vi "bias.vi"(10 "Cluster":T3={"Numero di punti"=11, "fattore-measdelay"=65, "Periodo"=0.01, "source autorange gate"=FALSE, "Tensione gate"=1.0, "llimit-gate"=1.0, "Source Function Gate"=1, "Range Mode Gate"=0, "Autozero Mode Gate"=1, "tensione drain"=1.0, "limit-drain"=1.0, "Autozero Mode Drain"=1, "Source Function Drain"=1, "Range Mode Drain"=0, "source autorange drain"=FALSE, "range-gate"=0.01, "source_range_gate"=2.0, "range-drain"=0.01, "source_range_drain"=2.0} {"source_range_drain" items=["200 mV"=0.2, "2 V"=2.0, "20 V"=20.0, "200 V"=200.0]; "range-drain" items=["100 nA"=1e-07, "1 uA"=1e-06, "10 uA"=1e-05, "100 uA"=0.0001, "1 mA"=0.001, "10 mA"=0.01, "100 mA"=0.1, "1 A"=1.0]; "source_range_gate" items=["200 mV"=0.2, "2 V"=2.0, "20 V"=20.0, "200 V"=200.0]; "range-gate" items=["100 nA"=1e-07, "1 uA"=1e-06, "10 uA"=1e-05, "100 uA"=0.0001, "1 mA"=0.001, "10 mA"=0.01, "100 mA"=0.1, "1 A"=1.0]; "Range Mode Drain" items=["Auto Range Off", "Auto Range On", "Auto Range Follow Limit"]; "Source Function Drain" items=["Current", "Voltage"]; "Autozero Mode Drain" items=["Autozero Off", "Autozero Once", "Autozero Auto"]; "limit-drain" format="%#_13g"; "Autozero Mode Gate" items=["Autozero Off", "Autozero Once", "Autozero Auto"]; "Range Mode Gate" items=["Auto Range Off", "Auto Range On", "Auto Range Follow Limit"]; "Source Function Gate" items=["Current", "Voltage"]; "llimit-gate" format="%#_13g"; "Periodo" items=["500 uS", "1 mS", "2 mS", "5 mS", "10 mS", "20 mS", "50 mS", "100 mS", "200 mS", "500 mS", "1 S", "2 S", "5 S", "10 S", ""]}, 11 "Cluster 3":T2={"VISA resource name out"="USB0::0x05E6::0x2612::4671051::INSTR", "error out"={"status"=FALSE, "code"=0, "source"=""}}) -> (2 "Cluster 2":T1, 3 "output cluster":T2)   [LabVIEW 2025]
uses:
  <instrlib>/Keithley 2600 Series/Keithley 2600 Series.lvlib
panel:
  out "range misurato gate":string
  out "range misurato drain":string
  out "finestra di misura":dbl
  out "measdelay":dbl
  out "Frequenza di rete (Hz)":dbl
  # "Impostazioni connessione"
  # "SMUA"
  # "SMUB"
  # "tabella valori"
  # "Impostazioni funzione source"
  # "Impostazioni comuni"
  # "GATE"
  # "DRAIN"
  # "Impostazioni funzione misura"
  # "GATE"
  # "DRAIN"
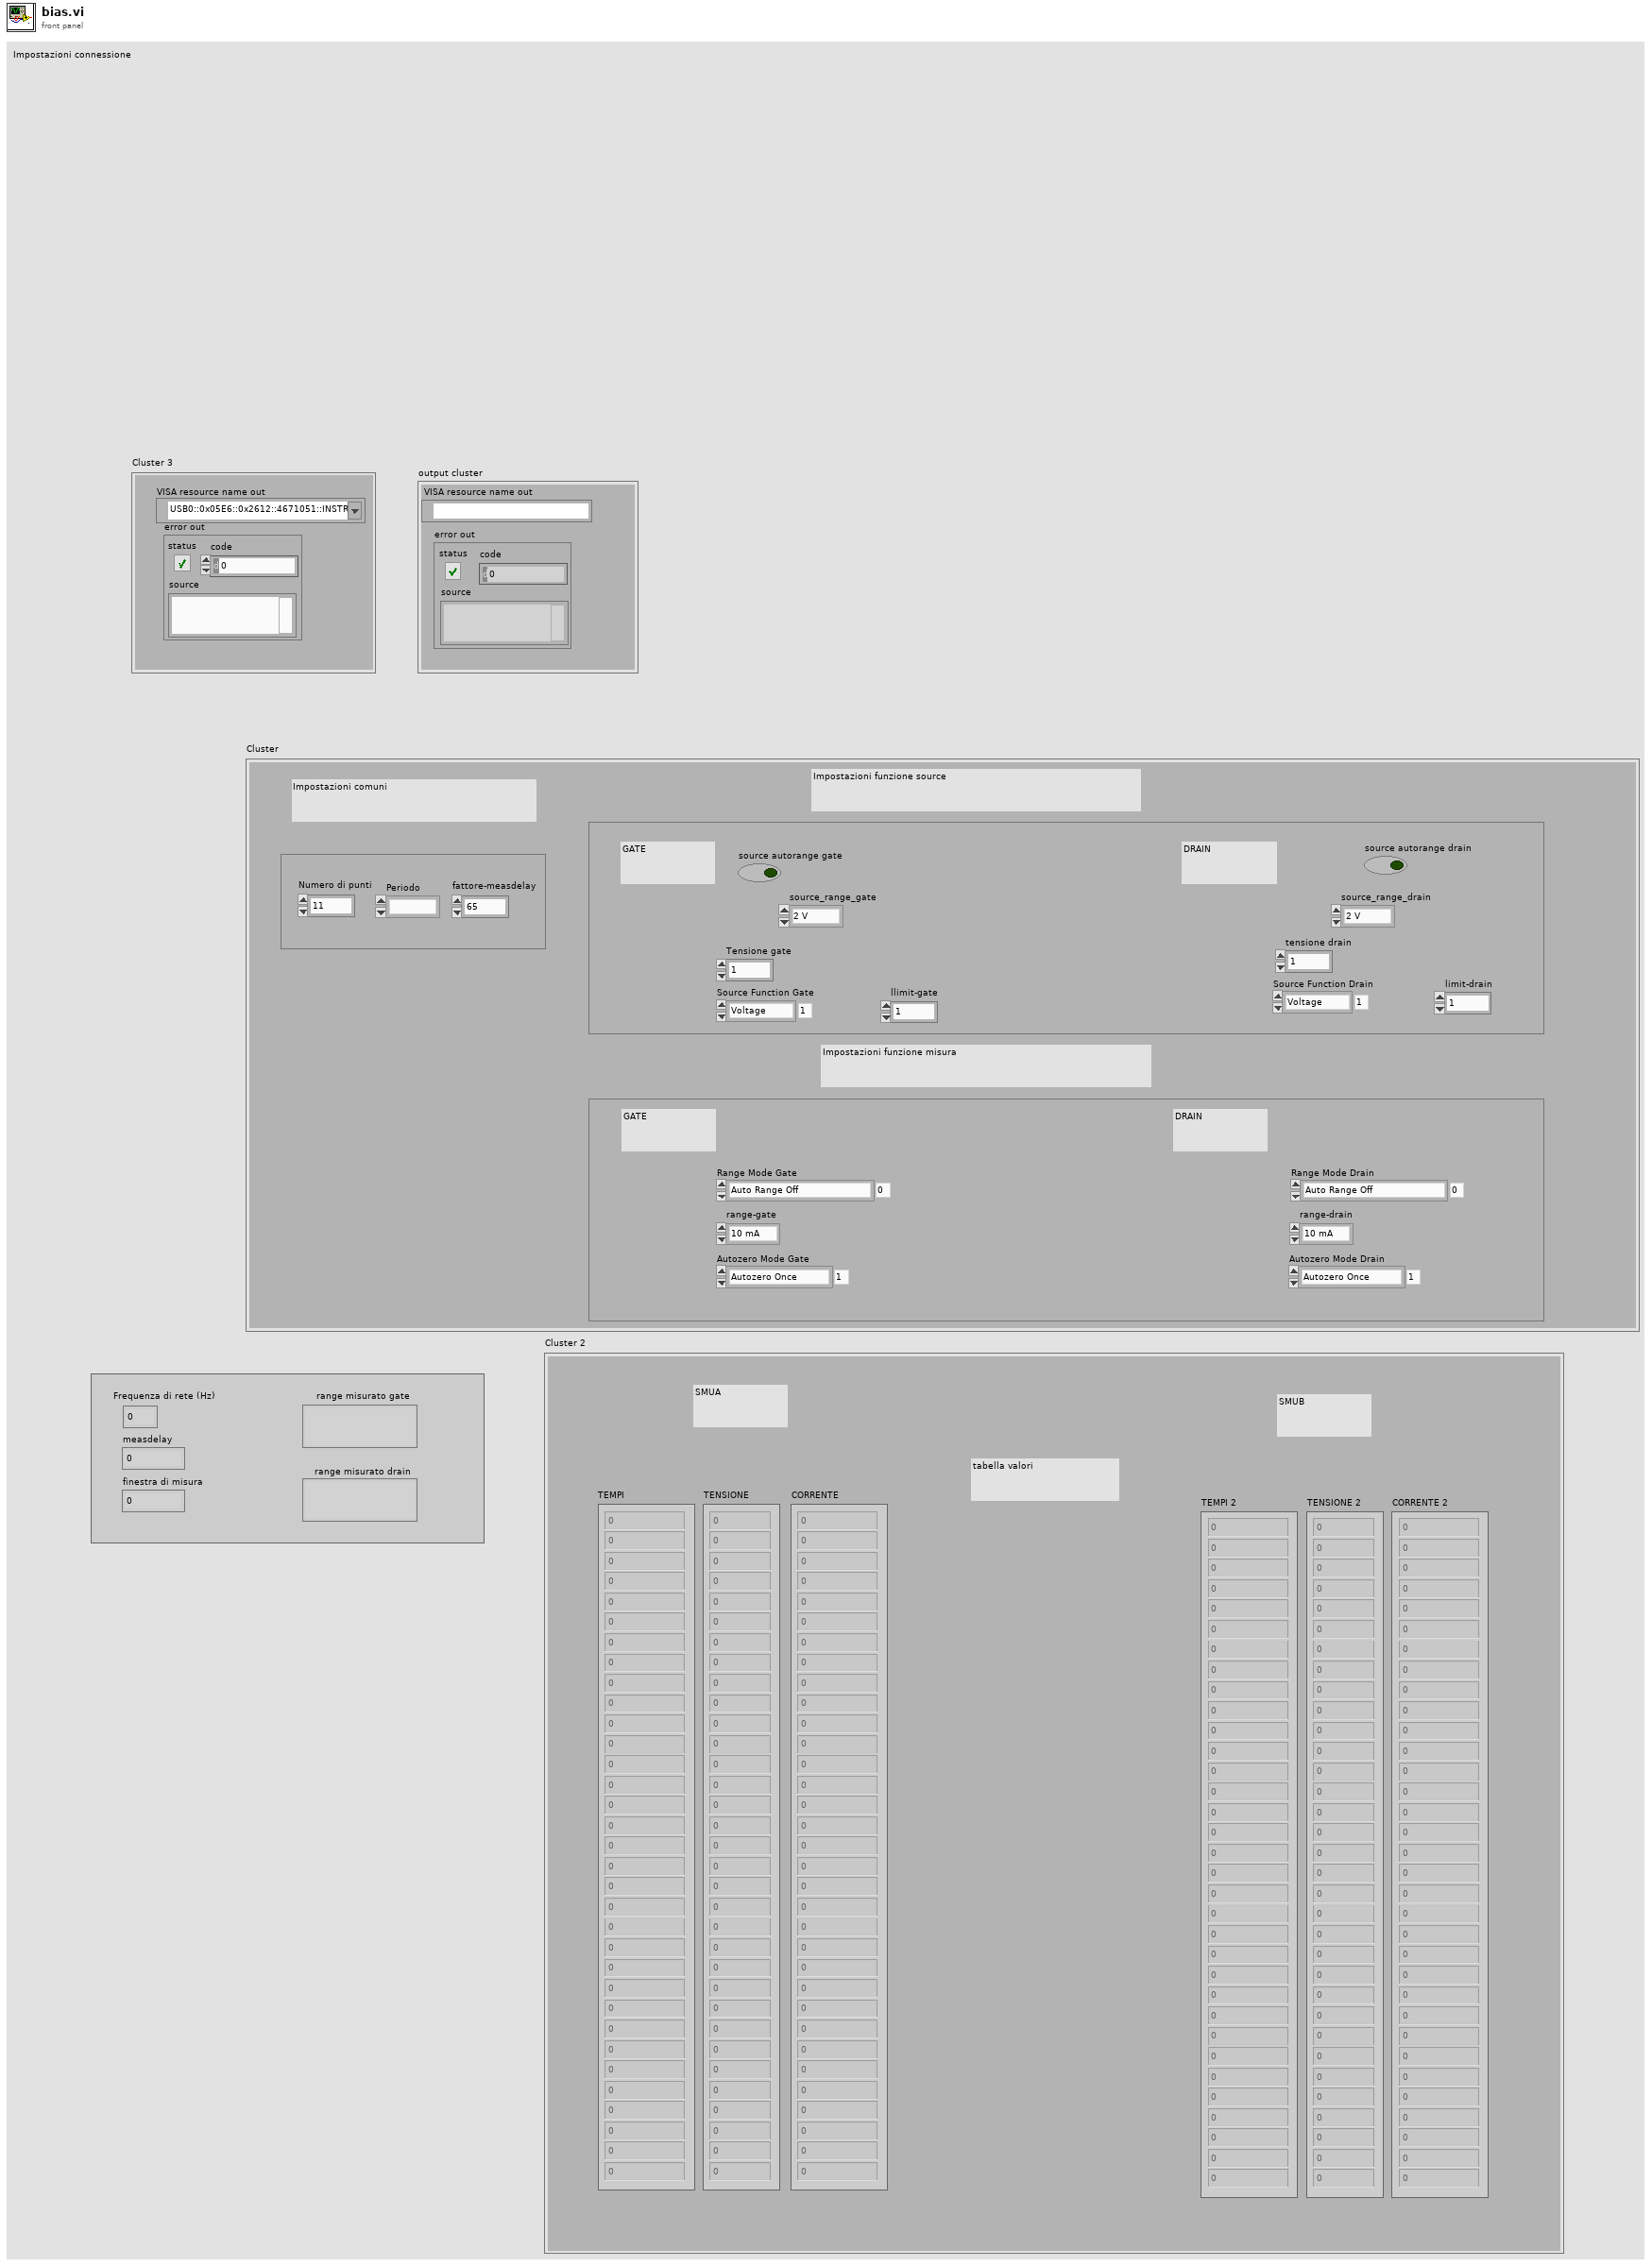
[diagram p1: front panel]
types:
  T1 = cluster{"CORRENTE":dbl[], "TENSIONE":dbl[], "TEMPI":dbl[], "CORRENTE 2":dbl[], "TENSIONE 2":dbl[], "TEMPI 2":dbl[]}
  T2 = cluster{"VISA resource name out":refnum<visa-resource-name>, "error out":errorcluster}
  T3 = cluster{"Numero di punti":i32, "fattore-measdelay":i32, "Periodo":ext, "source autorange gate":bool, "Tensione gate":dbl, "llimit-gate":dbl, "Source Function Gate":i32, "Range Mode Gate":i32, "Autozero Mode Gate":i32, "tensione drain":dbl, "limit-drain":dbl, "Autozero Mode Drain":i32, "Source Function Drain":i32, "Range Mode Drain":i32, "source autorange drain":bool, "range-gate":dbl, "source_range_gate":dbl, "range-drain":dbl, "source_range_drain":dbl}
  T4 = cluster{"CORRENTE":dbl[], "TENSIONE":dbl[], "TEMPI":dbl[], "CORRENTE":dbl[], "TENSIONE":dbl[], "TEMPI":dbl[]}
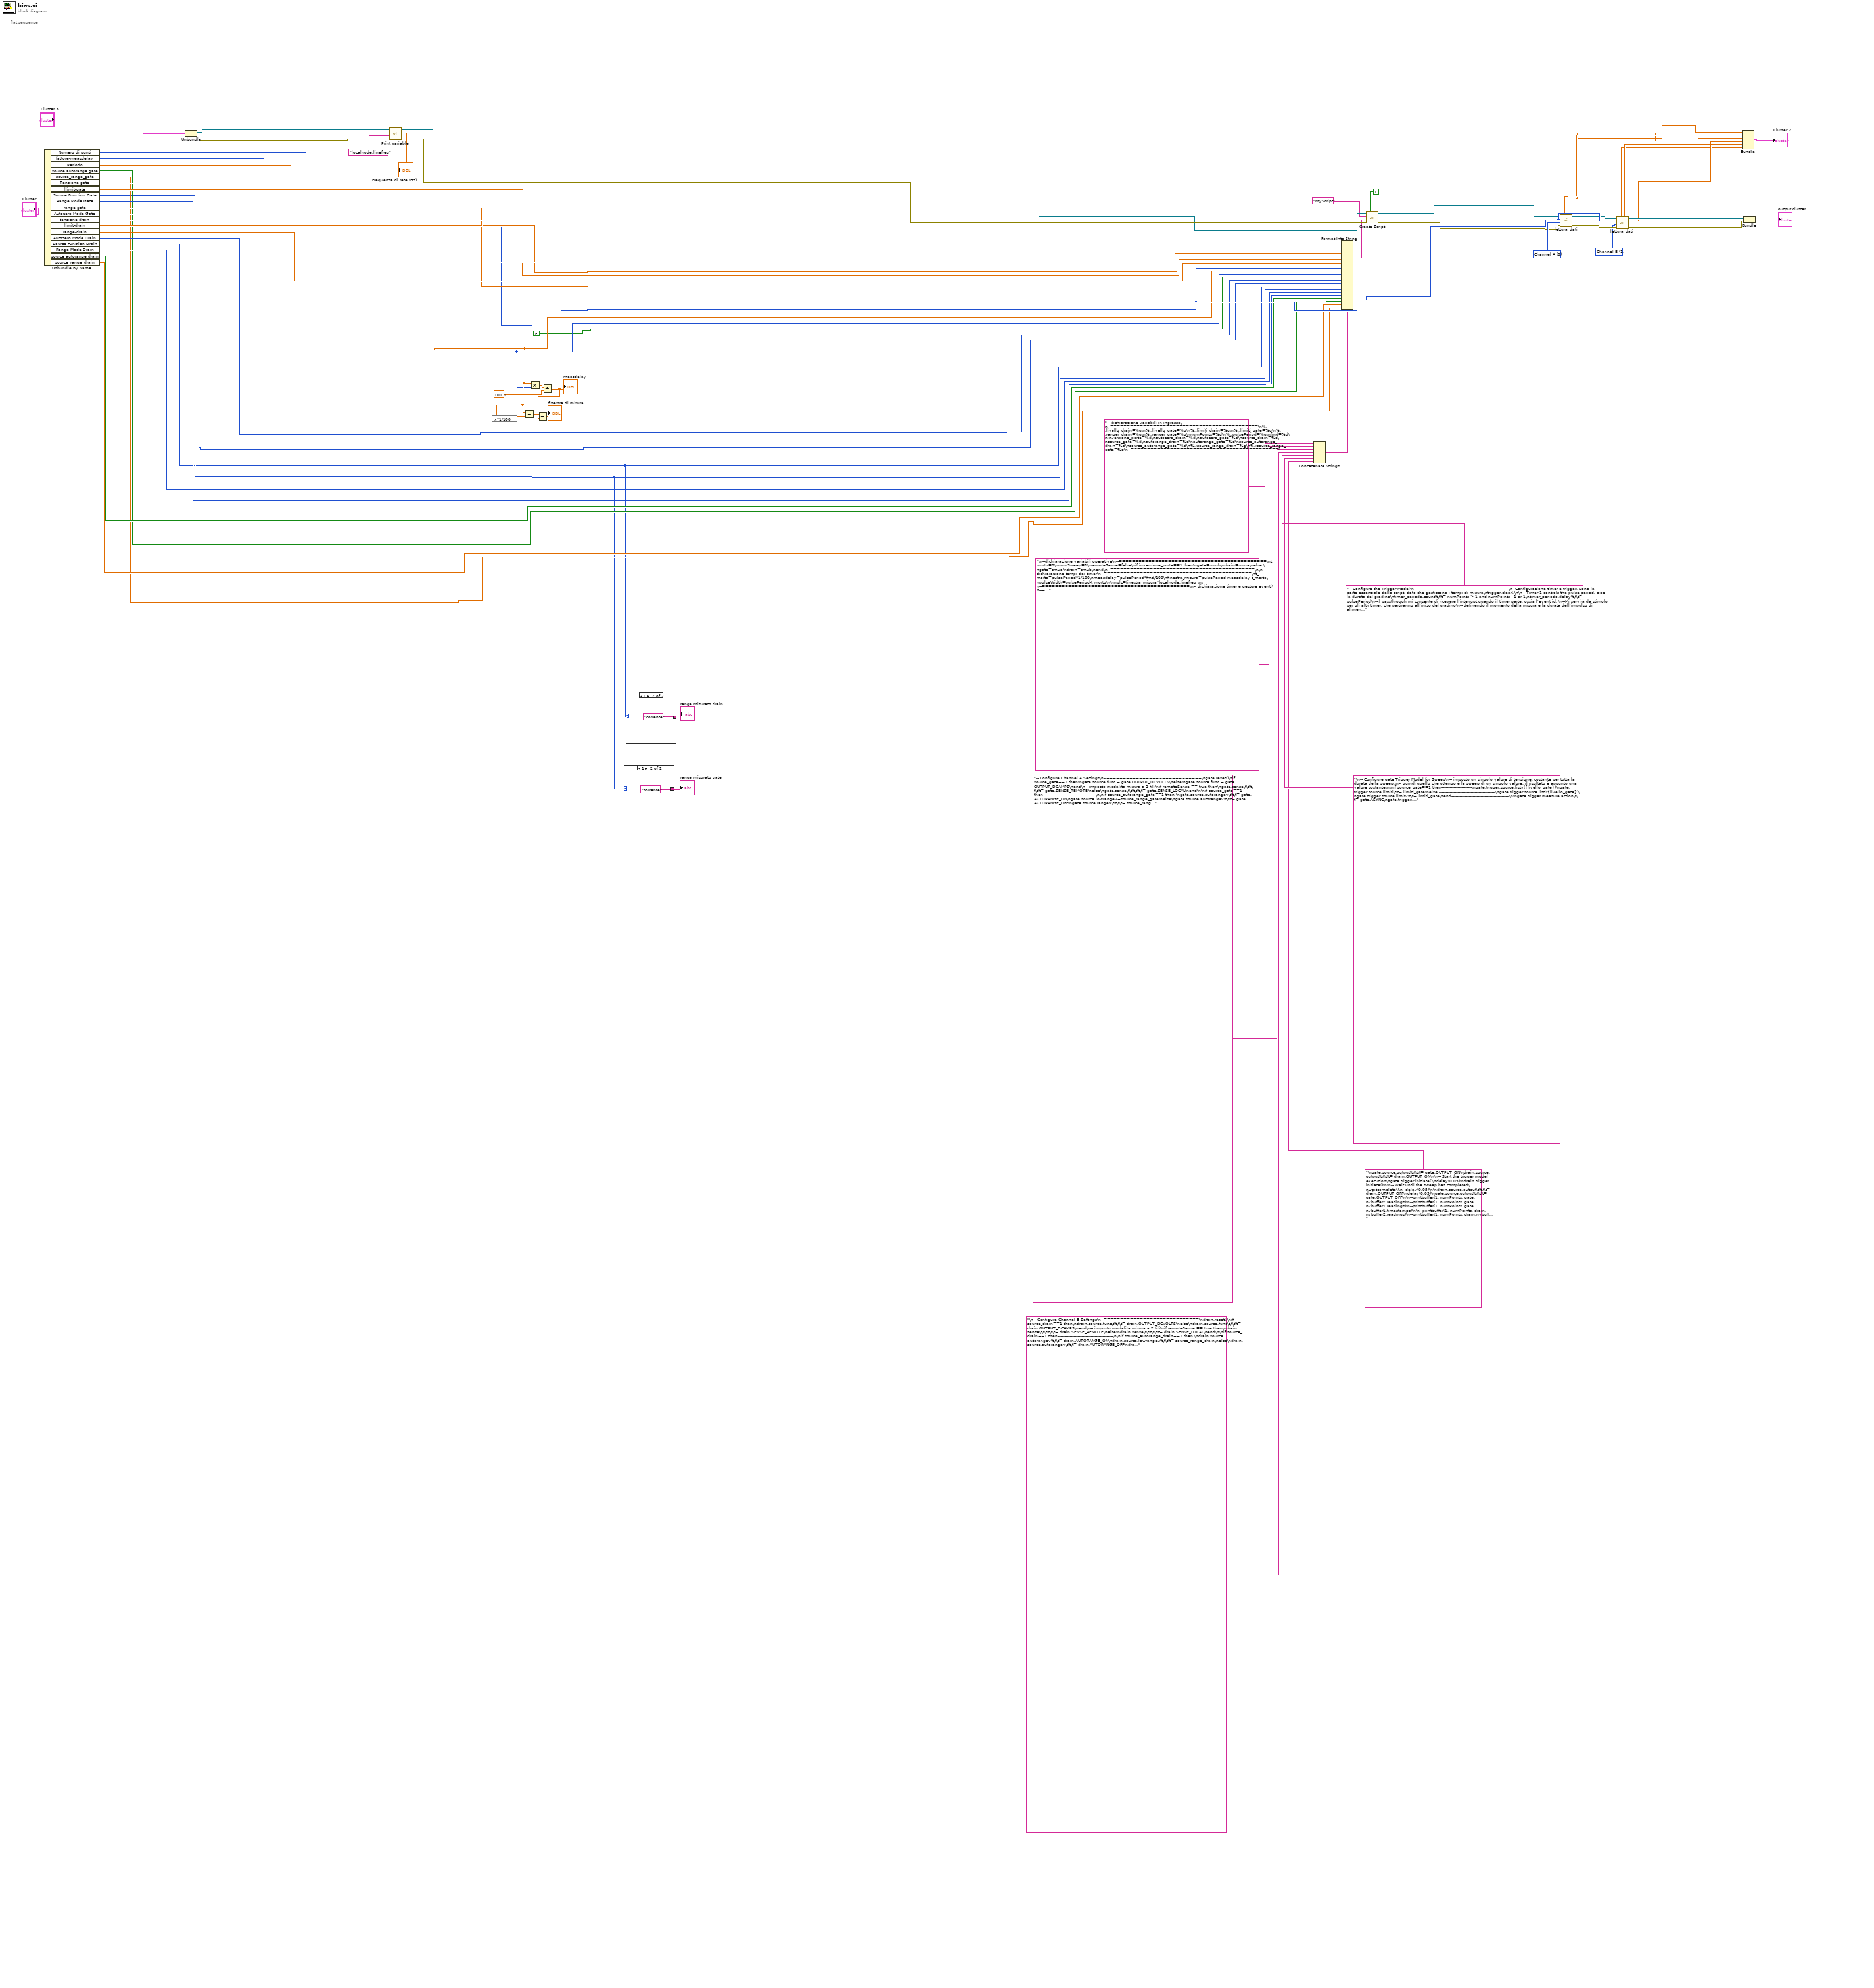
[diagram p0: block diagram]
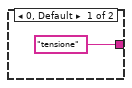
[diagram p2: hidden frame]
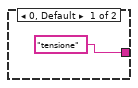
[diagram p3: hidden frame]
diagram:
  n1 = flat-sequence {
    frame #0 {
      w13 = 1 items=["Channel A", "Channel B"] ("Source Measure Unit Channel (0: Channel A)")
      w18 = 0 items=["Channel A", "Channel B"] ("Source Measure Unit Channel (0: Channel A)")
      n2 = Unbundle By Name("Cluster") -> ("Numero di punti"=w47:i32, "fattore-measdelay"=w39:i32, "Periodo"=w40:ext, "source autorange gate"=w33:bool, "source_range_gate"=w31:dbl, "Tensione gate"=w52:dbl, "llimit-gate"=w50:dbl, "Source Function Gate"=w9:i32, "Range Mode Gate"=w35:i32, "range-gate"=w48:dbl, "Autozero Mode Gate"=w37:i32, "tensione drain"=w53:dbl, "limit-drain"=w51:dbl, "range-drain"=w49:dbl, "Autozero Mode Drain"=w38:i32, "Source Function Drain"=w8:i32, "Range Mode Drain"=w36:i32, "source autorange drain"=w34:bool, "source_range_drain"=w32:dbl)
      n3 = Unbundle("Cluster 3") -> ("VISA resource name out"=w44:refnum<visa-resource-name>, "error out"=w43:errorcluster)
      n4 = call <instrlib>:"Print Variable.vi"("error in (no error)"=w43, "Variable Name"="localnode.linefreq", "VISA resource name"=w44) -> ("error out"=w55:errorcluster, "Number"=→"Frequenza di rete (Hz)":dbl, "VISA resource name out"=w54:refnum<visa-resource-name>)  [unwired: 5 in, 1 out]
      n5 = expression code="x*1/100"(w40) -> (w59:ext)
      n6 = Subtract(x=w40, y=w59) -> (x-y=w58:ext)
      n7 = Multiply(x=w40, y=w39) -> (x*y=w61:ext)
      n8 = Divide(x=w61, y=100.0) -> (x/y=w57:ext)
      "measdelay" <- w57
      n9 = Subtract(x=w58, y=w57) -> (x-y=→"finestra di misura":ext)
      n10 = case shown="1" w9 {
        tunnel: ["tensione" "corrente"] -> w10
        frame 0, Default {
        }
        frame 1 {
        }
      }
      "range misurato gate" <- w10
      n11 = case shown="1" w8 {
        tunnel: ["tensione" "corrente"] -> w11
        frame 0, Default {
        }
        frame 1 {
        }
      }
      "range misurato drain" <- w11
      n12 = Concatenate Strings("-- dichiarazione variabili in ingresso\n--=============================================\n%.;livello_drain=%g\n%.;livello_gate=%g\n%.;limiti_drain=%g\n%.;limiti_gate=%g\n%.;rangei_drain=%g\n%.;rangei_gate=%g\nnumPoints=%d\n%.;pulsePeriod=%g\nfmd=%d\ninversione_porte=%d\nautozero_drain=%d\nautozero_gate=%d\nsource_drain=%d\nsource_gate=%d\nautorange_drain=%d\nautorange_gate=%d\nsource_autorange_drain=%d\nsource_autorange_gate=%d\n%.;source_range_drain=%g\n%.;source_range_gate=%g\n--=============================================", "\n--dichiarazione variabili operative\n--=============================================\nt_morto=0\nnumSweep=1\nremoteSense=false\nif inversione_porte==1 then\ngate=smub\ndrain=smua\nelse \ngate=smua\ndrain=smub\nend\n--============================================\n\n-- dichiarazione tempi dei timer\n--=============================================\nt_morto=pulsePeriod*1/100\nmeasdelay=pulsePeriod*fmd/100\nfinestra_misura=pulsePeriod-measdelay-t_morto\npulseWidth=pulsePeriod-t_morto\n\nnplc=finestra_misura*localnode.linefreq \n\n--=============================================\n-- dichiarazione timer e gestore eventi\n--=============================================\n-- Timer 1: timer periodo (larghezza gradino)\ntimer_periodo=trigger.timer[1]\n-- Timer 2: Timer ritardo misura\ntimer_misura=trigger.timer[2]\n-- Timer 3: Pulse Width Timer\ntimer_larghezza_impulso=trigger.timer[3]\n\n-- Gestore eventi 1: Event Blender per la partenza di iniziale di gate e l'aggiornamento di gate al trigger di drain\ngestore_avvio_gate=trigger.blender[1]\n--=============================================", "-- Configure Channel A Settings\n--=============================\ngate.reset()\nif source_gate==1 then\ngate.source.func = gate.OUTPUT_DCVOLTS\nelse\ngate.source.func = gate.OUTPUT_DCAMPS\nend\n-- imposto modalità misura a 2 fili\nif remoteSense == true then\ngate.sense\t\t\t\t\t\t= gate.SENSE_REMOTE\nelse\ngate.sense\t\t\t\t\t\t= gate.SENSE_LOCAL\nend\n\nif source_gate==1 then ---------------------------------------\n\nif source_autorange_gate==1 then \ngate.source.autorangev\t\t\t= gate.AUTORANGE_ON\ngate.source.lowrangev=source_range_gate\nelse\ngate.source.autorangev\t\t\t= gate.AUTORANGE_OFF\ngate.source.rangev\t\t\t\t= source_range_gate\nend \n\ngate.source.levelv\t\t\t\t= 0\n-- Set the DC bias limit.  This is not the limit used during the pulses. ma è il valore di idle della gate\ngate.source.limiti\t\t\t\t= limiti_gate\n\nelse------------------------\n\nif source_autorange_gate==1 then\ngate.source.autorangei\t\t\t= gate.AUTORANGE_ON\ngate.source.lowrangei=source_range_gate\nelse\ngate.source.autorangei\t\t\t= gate.AUTORANGE_OFF\ngate.source.rangei\t\t\t= source_range_gate\nend\n\ngate.source.leveli\t\t\t\t= 0\n-- Set the DC bias limit.  This is not the limit used during the pulses. ma è il valore di idle della gate\ngate.source.limitv\t\t\t\t= limiti_gate\nend --------------------------------------------------\n\n\n-- Disabling Auto-Ranging and Auto-Zero ensures accurate and consistent timing\n\nif autozero_gate==0 then\ngate.measure.autozero\t\t\t= gate.AUTOZERO_OFF\nelseif autozero_gate==1 then\ngate.measure.autozero\t\t\t= gate.AUTOZERO_ONCE\nelse\ngate.measure.autozero\t\t\t= gate.AUTOZERO_AUTO\nend\n\nif autorange_gate==0 then ------------------------\n\nif source_gate==1 then\ngate.measure.autorangei\t\t\t= gate.AUTORANGE_OFF\ngate.measure.rangei\t\t\t\t= rangei_gate\nelse\ngate.measure.autorangev\t\t\t= gate.AUTORANGE_OFF\ngate.measure.rangev\t\t\t\t= rangei_gate\nend\n\nelseif  autorange_gate==1 then -----------\n\nif source_gate==1 then\ngate.measure.autorangei\t\t\t= gate.AUTORANGE_ON\ngate.measure.lowrangei\t\t\t\t= rangei_gate\nelse\ngate.measure.autorangev\t\t\t= gate.AUTORANGE_ON\ngate.measure.lowrangev\t\t\t\t= rangei_gate\nend\n\nelse --------------------------\n\nend -------------------------------\n\ngate.measure.nplc\t\t\t\t= nplc\n-- A timer will be used to set the measure delay and synchronize the measurement\n-- between the two SMUs so set the built in delay to 0.\ngate.measure.delay\t\t\t\t= 0\n\n-- Prepare the Reading Buffers\ngate.nvbuffer1.clear()\ngate.nvbuffer1.collecttimestamps= 1\ngate.nvbuffer2.clear()\ngate.nvbuffer2.collecttimestamps = 1\n--=============================\n-- End Channel A Settings\n", "\n-- Configure Channel B Settings\n--=============================\ndrain.reset()\nif source_drain==1 then\ndrain.source.func\t\t\t\t= drain.OUTPUT_DCVOLTS\nelse\ndrain.source.func\t\t\t\t= drain.OUTPUT_DCAMPS\nend\n-- imposto modalità misura a 2 fili\nif remoteSense == true then\ndrain.sense\t\t\t\t\t\t= drain.SENSE_REMOTE\nelse\ndrain.sense\t\t\t\t\t\t= drain.SENSE_LOCAL\nend\n\nif source_drain==1 then------------------------------------------\n\nif source_autorange_drain==1 then \ndrain.source.autorangev\t\t\t= drain.AUTORANGE_ON\ndrain.source.lowrangev\t\t\t\t= source_range_drain\nelse\ndrain.source.autorangev\t\t\t= drain.AUTORANGE_OFF\ndrain.source.rangev\t\t\t\t=source_range_drain\nend\n\ndrain.source.levelv\t\t\t\t= 0\n-- Set the DC bias limit.  This is not the limit used during the pulses. ma è il valore di idle della smu\ndrain.source.limiti\t\t\t\t= limiti_drain\nelse----------------------------------------------------\nif source_autorange_drain==1 then \ndrain.source.autorangei\t\t\t= drain.AUTORANGE_ON\ndrain.source.lowrangei\t\t\t\t=source_range_drain\nelse\ndrain.source.autorangei\t\t\t= drain.AUTORANGE_OFF\ndrain.source.rangei\t\t\t\t=source_range_drain\nend\ndrain.source.leveli\t\t\t\t= 0\n-- Set the DC bias limit.  This is not the limit used during the pulses. ma è il valore di idle della smu\ndrain.source.limitv\t\t\t\t= limiti_drain\nend----------------------------------------------\n\n-- Disabling Auto-Ranging and Auto-Zero ensures accurate and consistent timing\n\nif autozero_drain==0 then\ndrain.measure.autozero\t\t\t= drain.AUTOZERO_OFF\nelseif autozero_drain==1 then\ndrain.measure.autozero\t\t\t= drain.AUTOZERO_ONCE\nelseif autozero_drain==2 then\ndrain.measure.autozero\t\t\t= drain.AUTOZERO_AUTO\nend\n\nif autorange_drain==0 then --------------------------------\n\nif source_drain==1 then\ndrain.measure.autorangei\t\t\t= drain.AUTORANGE_OFF\ndrain.measure.rangei\t\t\t\t= rangei_drain\nelse\ndrain.measure.autorangev\t\t\t= drain.AUTORANGE_OFF\ndrain.measure.rangev\t\t\t\t= rangei_drain\nend\n\n\n\nelseif  autorange_drain==1 then ----------------------------\n\nif source_drain==1 then\ndrain.measure.autorangei\t\t\t= drain.AUTORANGE_ON\ndrain.measure.lowrangei\t\t\t\t= rangei_drain\nelse\ndrain.measure.autorangev\t\t\t= drain.AUTORANGE_ON\ndrain.measure.lowrangev\t\t\t\t= rangei_drain\nend\n\nelse\n\nend --------------------------------------------------------------\n\ndrain.measure.nplc\t\t\t\t= nplc\n-- A timer will be used to set the measure delay and synchronize the measurement\n-- between the two SMUs so set the built in delay to 0.\ndrain.measure.delay\t\t\t\t= 0\n\n-- Prepare the Reading Buffers\ndrain.nvbuffer1.clear()\ndrain.nvbuffer1.collecttimestamps= 1\ndrain.nvbuffer2.clear()\ndrain.nvbuffer2.collecttimestamps= 1\n--=============================\n-- End Channel B Settings", "-- Configure the Trigger Model\n--============================\n--Configurazione timer e trigger. Sono la parte essenziale dello script, dato che gestiscono i tempi di misura\ntrigger.clear()\n\n-- Timer 1 controls the pulse period, cioè la durata del gradino\ntimer_periodo.count\t\t\t= numPoints > 1 and numPoints - 1 or 1\ntimer_periodo.delay\t\t\t= pulsePeriod\n--il passthrough mi consente di ricevere l'interrupt quando il timer parte, ossia l'event id. \n--Mi servirà da stimolo per gli altri timer, che partiranno all'inizo del gradino\n-- definendo il momento della misura e la durata dell'impulso di alimentazione\ntimer_periodo.passthrough\t= true\n-- il timer 1 parte quando la drain, in questo caso, inizia la sweep: cioè entra nello stato armed\ntimer_periodo.stimulus\t\t= drain.trigger.ARMED_EVENT_ID \n\n-- Timer 2 controls the measurement. il timer 2 gestisce il ritardo di misura. scaduto quello, inizia la finestra di misura\ntimer_misura.count\t\t\t= 1\ntimer_misura.delay\t\t\t= measdelay\n-- il passthrough è false perchè l'interrupt lo produrre alla fine. \n-- Scaduto il delay di misura, inizia la finestra di misura\ntimer_misura.passthrough\t= false\n--il timer 1 grazie al passthrough mi fa partire il timer 2 all'inizio del gradino\ntimer_misura.stimulus\t\t= timer_periodo.EVENT_ID \n\n-- Timer 3 controls the pulse width\ntimer_larghezza_impulso.count\t\t\t= 1\ntimer_larghezza_impulso.delay\t\t\t= pulseWidth\n-- il passthrough è false perchè l'interrupt me lo produce alla fine, perchè \ntimer_larghezza_impulso.passthrough\t= false\n--il timer 1 grazie al passthrough mi fa partire il timer 3 all'inizio del gradino\ntimer_larghezza_impulso.stimulus\t\t= timer_periodo.EVENT_ID", "\n-- Configure gate Trigger Model for Sweep\n-- imposto un singolo valore di tensione, costante per tutta la durata della sweep.\n-- quindi quello che ottengo è la sweep di un singolo valore. il risultato è appunto una valore costante\n\nif source_gate==1 then-----------------------\ngate.trigger.source.listv({livello_gate})\ngate.trigger.source.limiti\t\t= limiti_gate\nelse -------------------------------------------\ngate.trigger.source.listi({livello_gate})\ngate.trigger.source.limitv\t\t= limiti_gate\nend--------------------------------------------\n\ngate.trigger.measure.action\t\t= gate.ASYNC\ngate.trigger.measure.iv(gate.nvbuffer1, gate.nvbuffer2)\n--fine impulso: se voglio una dc sweep, anzichè mandare in idle l'uscita, la tengo costante\ngate.trigger.endpulse.action\t= gate.SOURCE_HOLD\n-- endsweep mi dice cosa fare quando finisce l'operazione sweep\ngate.trigger.endsweep.action\t= gate.SOURCE_HOLD\ngate.trigger.arm.count = 1\ngate.trigger.count\t\t\t\t= numSweep\n-- arm sweep indica quanto sweep deve fare \ndrain.trigger.arm.stimulus\t\t= 0\n\n\n--event blender per la partenza\ngestore_avvio_gate.orenable = true\ngestore_avvio_gate.stimulus[1] = gate.trigger.ARMED_EVENT_ID\ngestore_avvio_gate.stimulus[2] = drain.trigger.ARMED_EVENT_ID \n\n--dico quali stimoli/timer attivano le azioni\ngate.trigger.source.stimulus = gestore_avvio_gate.EVENT_ID \ngate.trigger.measure.stimulus\t= timer_misura.EVENT_ID\ngate.trigger.endpulse.stimulus\t= drain.trigger.SWEEP_COMPLETE_EVENT_ID\n\ngate.trigger.source.action\t\t= gate.ENABLE\n\n-- Configure drain Trigger Model for Sweep\nif source_drain==1 then------------------------\ndrain.trigger.source.listv({livello_drain})\ndrain.trigger.source.limiti\t\t= limiti_drain\nelse---------------------------------------------\ndrain.trigger.source.listi({livello_drain})\ndrain.trigger.source.limitv\t\t= limiti_drain\nend---------------------------------------------\n\ndrain.trigger.measure.action\t\t= drain.ENABLE\ndrain.trigger.measure.iv(drain.nvbuffer1, drain.nvbuffer2)\n--fine impulso: se voglio una dc sweep, anzichè mandare in idle l'uscita, la tengo costante\ndrain.trigger.endpulse.action\t= drain.SOURCE_HOLD\n-- endsweep mi dice cosa fare quando finisce l'operazione sweep\ndrain.trigger.endsweep.action\t= drain.SOURCE_HOLD\ndrain.trigger.arm.count = numSweep\n-- num punti sweep\ndrain.trigger.count\t\t\t\t= numPoints\n-- arm sweep indica quanto sweep deve fare\ndrain.trigger.arm.stimulus\t\t= 0\n--dico quali timer attivanzo le azioni\ndrain.trigger.source.stimulus\t= timer_periodo.EVENT_ID\ndrain.trigger.measure.stimulus\t= timer_misura.EVENT_ID\ndrain.trigger.endpulse.stimulus\t= timer_larghezza_impulso.EVENT_ID\ndrain.trigger.source.action\t\t= drain.ENABLE\n--==============================\n-- End Trigger Model Configuration", "\ngate.source.output\t\t\t\t= gate.OUTPUT_ON\ndrain.source.output\t\t\t\t= drain.OUTPUT_ON\n\n-- Start the trigger model execution\ngate.trigger.initiate()\ndelay(0.05)\ndrain.trigger.initiate()\n\n-- Wait until the sweep has completed\nwaitcomplete()\n--delay(0.05)\n\ndrain.source.output\t\t\t\t= drain.OUTPUT_OFF\ndelay(0.05)\ngate.source.output\t\t\t\t= gate.OUTPUT_OFF\n\n--printbuffer(1, numPoints, gate.nvbuffer2.readings)\n--printbuffer(1, numPoints, gate.nvbuffer1.readings)\n--printbuffer(1, numPoints, gate.nvbuffer1.timestamps)\n\n--printbuffer(1, numPoints, drain.nvbuffer2.readings)\n--printbuffer(1, numPoints, drain.nvbuffer1.readings)\n--printbuffer(1, numPoints, drain.nvbuffer1.timestamps)") -> (w26:string)
      n13 = Format Into String(format string=w26, w53, w52, w51, w50, w49, w48, w47, w40, w39, FALSE ("inversione_porte"), w38, w37, w8, w9, w36, w35, w34, w33, w32, w31) -> (resulting string=w29:string)  [unwired: 2 in, 1 out]
      n14 = call <instrlib>:"Create Script.vi"("Auto Run (F: Disable)"=TRUE, "error in (no error)"=w55, "Source Code"=w29, "Script Variable"="myScript", "VISA resource name"=w54) -> ("error out"=w16:errorcluster, "VISA resource name out"=w17:refnum<visa-resource-name>)  [unwired: 5 in]
      n15 = call "lettura_dati.vi"("error in (no error)"=w16, "Source Measure Unit Channel (0: Channel A)"=w18, "End Index (1)"=w47, "VISA resource name"=w17) -> ("error out"=w15:errorcluster, "CORRENTE"=w5:dbl[], "VISA resource name out"=w14:refnum<visa-resource-name>, "TENSIONE"=w7:dbl[], "TEMPI"=w4:dbl[])  [unwired: 3 in]
      n16 = call "lettura_dati.vi"("error in (no error)"=w15, "Source Measure Unit Channel (0: Channel A)"=w13, "End Index (1)"=w47, "VISA resource name"=w14) -> ("error out"=w12:errorcluster, "CORRENTE"=w2:dbl[], "VISA resource name out"=w42:refnum<visa-resource-name>, "TENSIONE"=w6:dbl[], "TEMPI"=w1:dbl[])  [unwired: 3 in]
      n17 = Bundle("CORRENTE"=w5, "TENSIONE"=w7, "TEMPI"=w4, "CORRENTE"=w2, "TENSIONE"=w6, "TEMPI"=w1) -> (→"Cluster 2":T4)  [unwired: 1 in]
      n18 = Bundle("VISA resource name out"=w42, "error out"=w12) -> (→"output cluster":T2)  [unwired: 1 in]
    }
  }
